vi "DataLog Linearly Interpolate Points.vi"(1 "times":dbl[](array[numeric]) format="%<%H:%M:%S%2u\n%Y/%m/%d>T", 2 "points":T1[](array[typedef]) {"value" format="%.3e"; "time" format="%<%H:%M:%S%2u\n%Y/%m/%d>T"}) -> (0 "interpolated values":dbl[](array[numeric]))   [LabVIEW 2012]
doc: "Serves the interpolation of number tags of \"sample\" temporal type. Linearly interpolate points at the given times (which need not be ordered). The timestamps of the points are assumed to increase monotonically. Interpolation at a time that lies outside the time range of the points results in a NaN value. The algorithm scales as O(T*log(P)) where T is the number of times to interpolate at and P the number of points."
uses:
  typedefs/clusters/t_DataLog Point.ctl
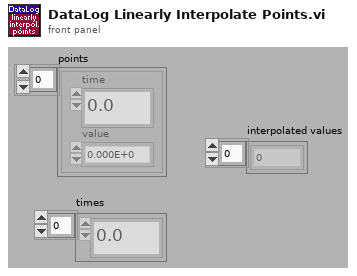
[diagram p1: front panel]
types:
  T1 = typedef "t_DataLog Point.ctl" = cluster{"time":dbl, "value":dbl}
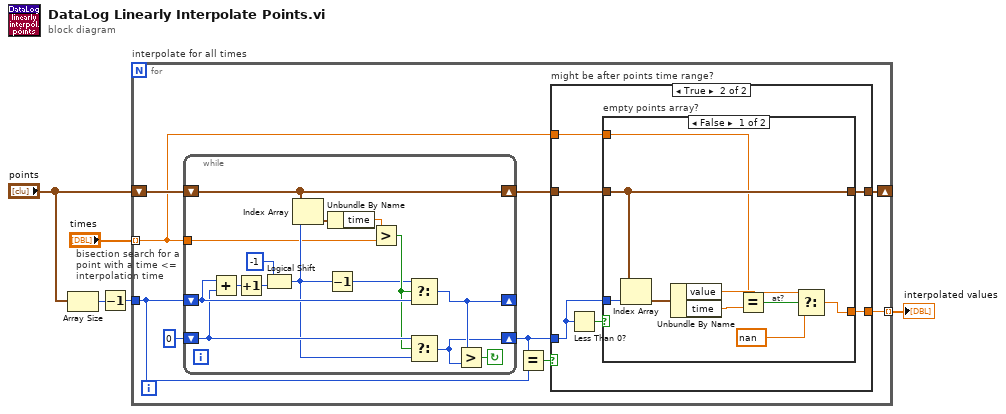
[diagram p0: block diagram]
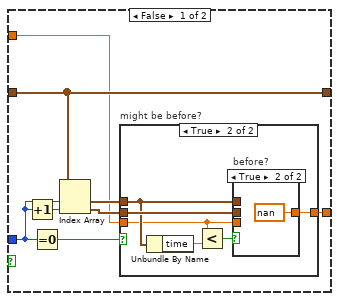
[diagram p2: hidden frame]
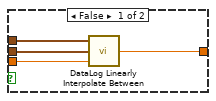
[diagram p3: hidden frame]
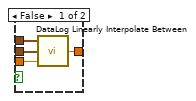
[diagram p4: hidden frame]
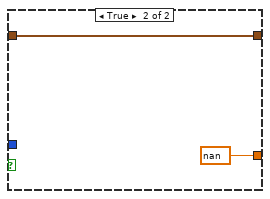
[diagram p5: hidden frame]
diagram:
  n1 = Array Size(array="points") -> (size(s)=w5:i32)
  n2 = Decrement(x=w5) -> (x-1=w4:i32)
  n3 = for "interpolate for all times" {
    tunnel: w4 -> [w13]
    tunnel: "times" -> [w11] mode=indexing
    shift-right: [w8] -> _
    shift-left: "points" -> [w12]
    tunnel: [w9] -> w1 mode=indexing
    n4 = while "bisection search for a point with a time <= interpolation time" {
      shift-right: [w61] -> w6
      shift-left: 0 -> [w68]
      shift-right: [w67] -> _
      shift-left: w13 -> [w69]
      tunnel: w11 -> [w58]
      shift-right: [w55] -> w10
      shift-left: w12 -> [w55]
      stop <- w66 continue-if-true
      n5 = Add(x=w69, y=w68) -> (x+y=w64:i32)
      n6 = Increment(x=w64) -> (x+1=w59:i32)
      n7 = Logical Shift(y=-1, x=w59) -> (x << y=w62:i32)
      n8 = Index Array(array=w55, index=w62) -> (element=w57:T1)
      n9 = Decrement(x=w62) -> (x-1=w60:i32)
      n10 = Unbundle By Name(w57) -> ("time"=w56:dbl)
      n11 = Greater?(x=w56, y=w58) -> (0:w65:bool)
      n12 = Select(t=w60, s=w65, f=w69) -> (s? t:f=w67:i32)
      n13 = Select(t=w68, s=w65, f=w62) -> (s? t:f=w61:i32)
      n14 = Greater?(x=w67, y=w61) -> (0:w66:bool)
    }
    n15 = Equal?(x=w6, y=w13) -> (x = y?=w7:bool)
    n16 = case "might be after points time range?" shown="True" w7 {
      tunnel: w6 -> [w16 w38]
      tunnel: w11 -> [w17 w40]
      tunnel: w10 -> [w21 w43]
      tunnel: [w22 w42] -> w9
      tunnel: [w21 w41] -> w8
      frame False {
        n17 = Increment(x=w16) -> (x+1=w19:i32)
        n18 = Equal To 0?(x=w16) -> (x = 0?=w15:bool)
        n19 = Index Array(array=w21, index #1=w16, index #2=w19) -> (element #1=w18:T1, element #2=w20:T1)
        n20 = case "might be before?" shown="True" w15 {
          tunnel: [w26 w32] -> w22
          tunnel: w20 -> [w25 w31]
          tunnel: w18 -> [w24 w30]
          tunnel: w17 -> [w23 w28]
          frame False {
            n21 = call "DataLog Linearly Interpolate Between.vi"("at"=w23, "point 2"=w25, "point 1"=w24) -> ("value"=w26:dbl)
          }
          frame True {
            n22 = Unbundle By Name(w30) -> ("time"=w29:dbl)
            n23 = Less?(x=w28, y=w29) -> (x < y?=w27:bool)
            n24 = case "before?" shown="True" w27 {
              tunnel: [w36 nan ("value")] -> w32
              tunnel: w31 -> [w35 _]
              tunnel: w30 -> [w34 _]
              tunnel: w28 -> [w33 _]
              frame False {
                n25 = call "DataLog Linearly Interpolate Between.vi"("at"=w33, "point 2"=w35, "point 1"=w34) -> ("value"=w36:dbl)
              }
              frame True {
              }
            }
          }
        }
      }
      frame True {
        n26 = Less Than 0?(x=w38) -> (x < 0?=w39:bool)
        n27 = case "empty points array?" shown="False" w39 {
          tunnel: w43 -> [w45 w54]
          tunnel: w38 -> [w52 _]
          tunnel: [w46 nan ("value")] -> w42
          tunnel: [w45 w54] -> w41
          tunnel: w40 -> [w44 _]
          frame False {
            # "at?"
            n28 = Index Array(array=w45, index=w52) -> (element=w51:T1)
            n29 = Unbundle By Name(w51) -> ("value"=w48:dbl, "time"=w50:dbl)
            n30 = Equal?(x=w44, y=w50) -> (x = y?=w49:bool)
            n31 = Select(t=w48, s=w49, f=nan ("value")) -> (s? t:f=w46:dbl)
          }
          frame True {
          }
        }
      }
    }
  }
  "interpolated values" <- w1
